vi "Write State.vi"(8 "error in (no error)":errorcluster, 10 "Set":T1, 11 "SimFlatShutt in":refnum<class "SimFlatShutt.lvclass">) -> (0 "error out":errorcluster, 3 "SimFlatShutt out":refnum<class "SimFlatShutt.lvclass">)   [LabVIEW 2016, in "SimFlatShutt.lvclass"]
uses:
  SimFlatShutt.lvclass
  Controls/Shutter States.ctl
  Shutter.lvclass
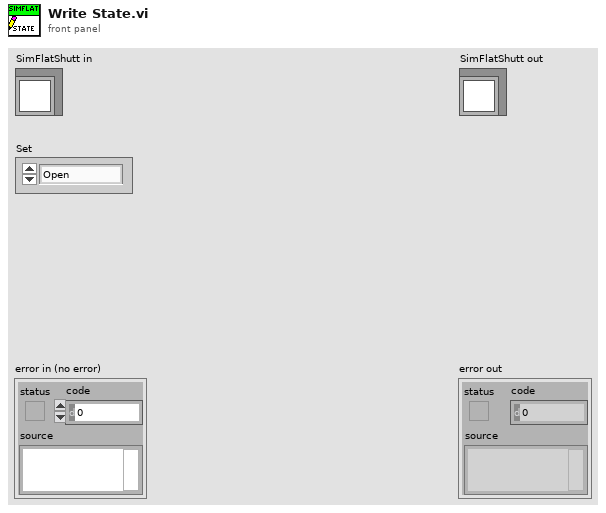
[diagram p1: front panel]
types:
  T1 = typedef "Shutter States.ctl" = enum16{"Open", "Close", "Wait", "Off", "Arm", "Idle"}
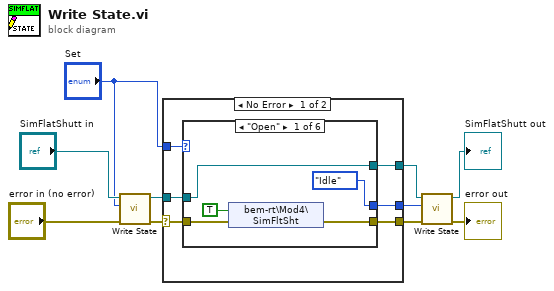
[diagram p0: block diagram]
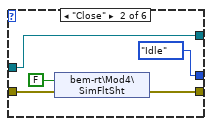
[diagram p2: hidden frame]
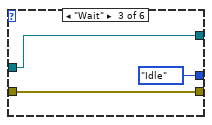
[diagram p3: hidden frame]
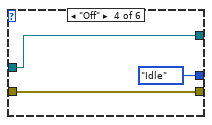
[diagram p4: hidden frame]
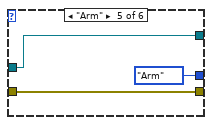
[diagram p5: hidden frame]
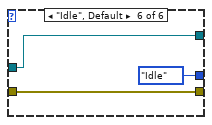
[diagram p6: hidden frame]
diagram:
  n1 = call-parent "Write State.vi"("error in (no error)"="error in (no error)", "Set"="Set", "Shutter in"="SimFlatShutt in") -> ("error out"=w3:errorcluster, "Shutter out"=w2:refnum<class "SimFlatShutt.lvclass">)  [unwired: 7 in]
  n2 = case shown="No Error" w3 {
    selector: w3 -> [w11 w41]
    tunnel: "Set" -> [w16 w39]
    tunnel: w2 -> [w15 w40]
    tunnel: [w14 w41] -> w8
    tunnel: [w13 w40] -> w7
    tunnel: [w12 w39] -> w6
    frame No Error {
      n3 = case shown="\"Open\"" w16 {
        tunnel: w11 -> [w20 w25 w29 w32 w35 w38]
        tunnel: [w17 w23 w29 w32 w35 w38] -> w14
        tunnel: w15 -> [w18 w22 w28 w31 w34 w37]
        tunnel: [w18 w22 w28 w31 w34 w37] -> w13
        tunnel: [Shutter_States."Idle" ("Set") Shutter_States."Idle" ("Set") Shutter_States."Idle" ("Set") Shutter_States."Idle" ("Set") Shutter_States."Arm" ("Set") Shutter_States."Idle" ("Set")] -> w12
        frame "Open" {
          n4 = shared-variable "bem-rt\\Mod4\\SimFltSht"(TRUE ("ExtFltSht"), error in=w20) -> (error out=w17:errorcluster)
        }
        frame "Close" {
          n5 = shared-variable "bem-rt\\Mod4\\SimFltSht"(FALSE ("ExtFltSht"), error in=w25) -> (error out=w23:errorcluster)
        }
        frame "Wait" {
        }
        frame "Off" {
        }
        frame "Arm" {
        }
        frame "Idle", Default {
        }
      }
    }
    frame Error {
    }
  }
  n6 = call-parent "Write State.vi"("error in (no error)"=w8, "Set"=w6, "Shutter in"=w7) -> ("error out"=→"error out":errorcluster, "Shutter out"=→"SimFlatShutt out":refnum<class "SimFlatShutt.lvclass">)  [unwired: 7 in]
